vi "Barcos.vi"() -> ()   [LabVIEW 2018]
uses:
  af593242-30fc-4f16-b0cf-da85950422bf.vi
  3aae2fef-4c67-42df-add4-2f8851009a90.vi
panel:
  in  "stop":bool
  in  "Clean":bool
  in  "Start":bool
  out "Barcos":bool[](array[boolean])
  in  "Barcos Conf.":dbl[](array[numeric])
  in  "Array":bool[][](array[boolean])
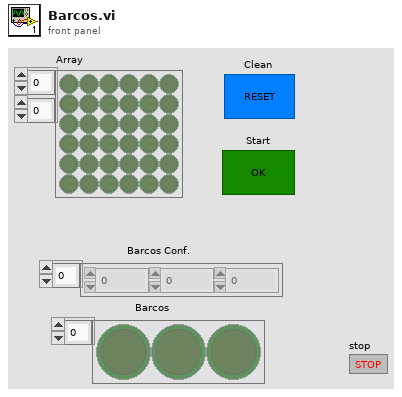
[diagram p1: front panel]
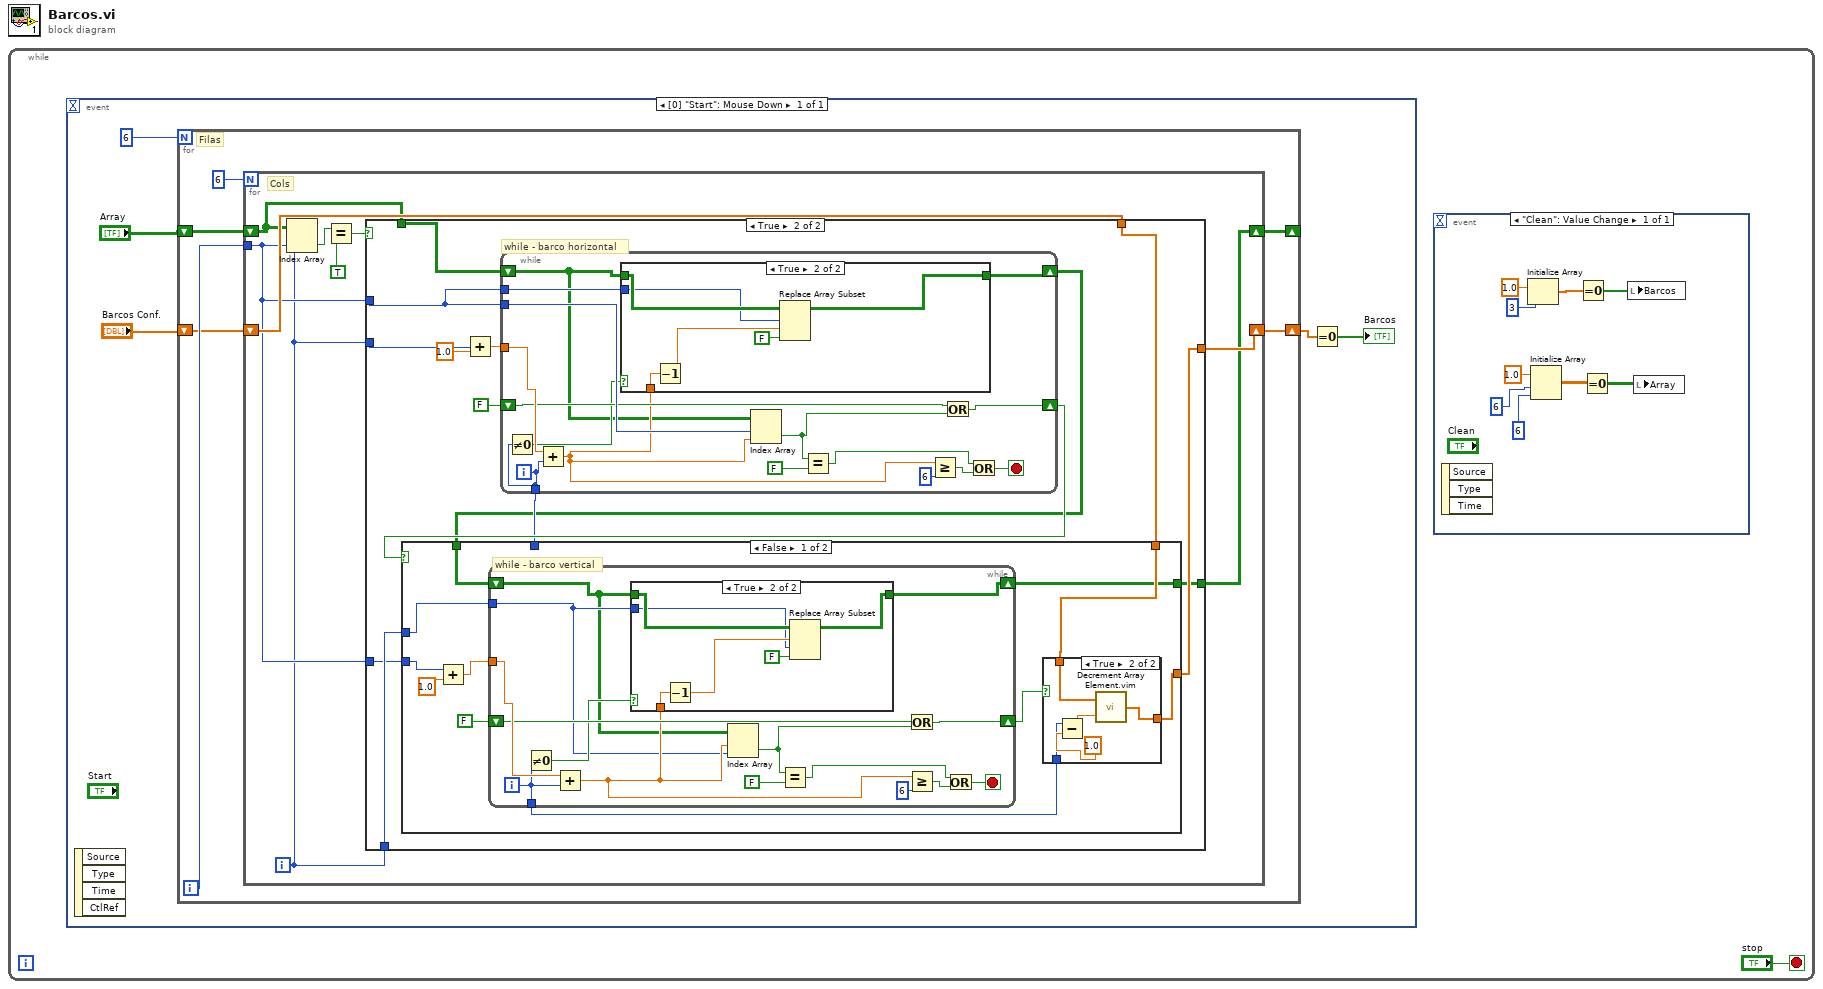
[diagram p0: block diagram]
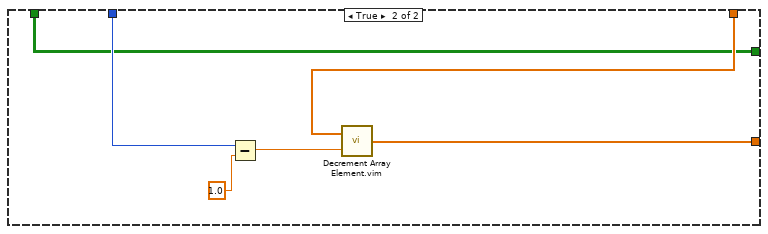
[diagram p5: hidden frame]
diagram:
  n1 = while {
    stop <- "stop" stop-if-true
    n2 = event shown="[0] \"Start\": Mouse Down" {
      selector: _ -> [_]
      dyn-events: _ -> [_]
      timeout: _ -> [_]
      event "Start": Mouse Down {
        n3 = event-data() -> ()  [unwired: 1 in, 4 out]
        n4 = for {
          N: 6 -> [_]
          shift-right: [w17] -> _
          shift-left: "Array" -> [w21]
          shift-right: [w18] -> w12
          shift-left: "Barcos Conf." -> [w19]
          i -> [w20]
          # "Filas"
          n5 = for {
            N: 6 -> [_]
            tunnel: w20 -> [w25]
            shift-right: [w22] -> w17
            shift-left: w21 -> [w23]
            shift-right: [w27] -> w18
            shift-left: w19 -> [w26]
            i -> [w24]
            # "Cols"
            n6 = Index Array(array=w23, index (row)=w25, index (col)=w24) -> (element=w29:bool)
            n7 = Equal?(x=w29, y=TRUE) -> (x = y?=w28:bool)
            n8 = case shown="True" w28 {
              tunnel: w25 -> [_ w46]
              tunnel: w24 -> [_ w40]
              tunnel: w23 -> [w32 w43]
              tunnel: w26 -> [w31 w39]
              tunnel: w25 -> [_ w35]
              tunnel: [w31 w37] -> w27
              tunnel: w24 -> [_ w36]
              tunnel: [w32 w33] -> w22
              frame False {
              }
              frame True {
                # "while - barco horizontal"
                n9 = Add(x=w40, y=1.0) -> (x+y=w42:dbl)
                n10 = while {
                  tunnel: w46 -> [w107]
                  tunnel: w42 -> [w106]
                  tunnel: w46 -> [w102]
                  shift-right: [w101] -> w34
                  shift-left: w43 -> [w93]
                  shift-right: [w94] -> w45
                  shift-left: FALSE -> [w100]
                  tunnel: [w95] -> w44
                  i -> [w95]
                  stop <- w105 stop-if-true
                  n11 = Not Equal To 0?(x=w95) -> (x != 0?=w99:bool)
                  n12 = Add(x=w106, y=w95) -> (x+y=w96:dbl)
                  n13 = case shown="True" w99 {
                    tunnel: w93 -> [w108 w114]
                    tunnel: w102 -> [_ w113]
                    tunnel: [w108 w111] -> w101
                    tunnel: w96 -> [_ w110]
                    frame False {
                    }
                    frame True {
                      n14 = Decrement(x=w110) -> (x-1=w109:dbl)
                      n15 = Replace Array Subset(array=w114, new element=FALSE ("new element/subarray"), index (row)=w113, index (col)=w109) -> (w111:bool[][])
                    }
                  }
                  n16 = Index Array(array=w93, index (row)=w107, index (col)=w96) -> (element=w92:bool)
                  n17 = Equal?(x=w92, y=FALSE) -> (x = y?=w98:bool)
                  n18 = Greater Or Equal?(x=w96, y=6) -> (x >= y?=w104:bool)
                  n19 = Or(x=w100, y=w92) -> (x .or. y?=w94:bool)
                  n20 = Or(x=w98, y=w104) -> (x .or. y?=w105:bool)
                }
                n21 = case shown="False" w45 {
                  tunnel: w39 -> [w52 w91]
                  tunnel: w44 -> [_ w87]
                  tunnel: [w51 w88] -> w37
                  tunnel: w36 -> [w53 _]
                  tunnel: w35 -> [w50 _]
                  tunnel: w34 -> [w48 w86]
                  tunnel: [w47 w86] -> w33
                  frame False {
                    # "while - barco vertical"
                    n22 = Add(x=w50, y=1.0) -> (x+y=w49:dbl)
                    n23 = while {
                      tunnel: w49 -> [w78]
                      shift-right: [w64] -> w47
                      shift-left: w48 -> [w66]
                      shift-right: [w67] -> w57
                      shift-left: FALSE -> [w74]
                      tunnel: [w70] -> w56
                      tunnel: w53 -> [w68]
                      i -> [w70]
                      stop <- w77 stop-if-true
                      n24 = Not Equal To 0?(x=w70) -> (x != 0?=w73:bool)
                      n25 = Add(x=w78, y=w70) -> (x+y=w69:dbl)
                      n26 = case shown="True" w73 {
                        tunnel: w66 -> [w79 w85]
                        tunnel: w69 -> [_ w83]
                        tunnel: w68 -> [_ w81]
                        tunnel: [w79 w80] -> w64
                        frame False {
                        }
                        frame True {
                          n27 = Decrement(x=w83) -> (x-1=w82:dbl)
                          n28 = Replace Array Subset(array=w85, new element=FALSE ("new element/subarray"), index (row)=w82, index (col)=w81) -> (w80:bool[][])
                        }
                      }
                      n29 = Index Array(array=w66, index (row)=w69, index (col)=w68) -> (element=w65:bool)
                      n30 = Equal?(x=w65, y=FALSE) -> (x = y?=w72:bool)
                      n31 = Or(x=w74, y=w65) -> (x .or. y?=w67:bool)
                      n32 = Greater Or Equal?(x=w69, y=6) -> (x >= y?=w76:bool)
                      n33 = Or(x=w72, y=w76) -> (x .or. y?=w77:bool)
                    }
                    n34 = case shown="True" w57 {
                      tunnel: w52 -> [w58 w63]
                      tunnel: w56 -> [_ w60]
                      tunnel: [w58 w59] -> w51
                      frame False {
                      }
                      frame True {
                        n35 = Subtract(x=w60, y=1.0) -> (x-y=w62:dbl)
                        n36 = call "Decrement Array Element.vim"("index"=w62, "array in"=w63) -> ("array out"=w59:dbl[])
                      }
                    }
                  }
                  frame True {
                    n37 = Subtract(x=w87, y=1.0) -> (x-y=w90:dbl)
                    n38 = call "Decrement Array Element.vim"("index"=w90, "array in"=w91) -> ("array out"=w88:dbl[])
                  }
                }
              }
            }
          }
        }
        n39 = Equal To 0?(x=w12) -> (x = 0?=→"Barcos":bool[])
      }
    }
    n40 = event shown="[0] \"Clean\": Value Change" {
      selector: _ -> [_]
      dyn-events: _ -> [_]
      timeout: _ -> [_]
      event "Clean": Value Change {
        n41 = event-data() -> ()  [unwired: 1 in, 3 out]
        n42 = Initialize Array(1.0 ("element"), 3 ("dimension size")) -> (w8:dbl[])
        n43 = Initialize Array(1.0 ("element"), 6 ("dimension size"), 6 ("dimension size")) -> (w4:dbl[][])
        n44 = Equal To 0?(x=w8) -> (x = 0?=w7:bool[])
        n45 = Equal To 0?(x=w4) -> (x = 0?=w5:bool[][])
        n46 = local write "Barcos"(w7) -> ()
        n47 = local write "Array"(w5) -> ()
      }
    }
  }
